vi "ConsolidatedLaunchingCode.vi"(8 "error in (no error)":errorcluster, 9 "Timeout (s)":i32, 11 "PullBack":bool) -> (0 "error out":errorcluster)   [LabVIEW 2013]
uses:
  <vilib>/Rock Robotics/WPI/CAN/Jaguar/SubVIs/WPI_CANJaguar_StatusSelect.ctl
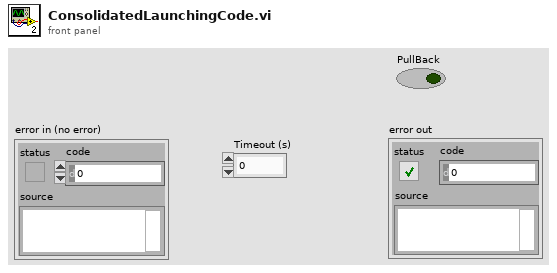
[diagram p1: front panel]
types:
  T1 = typedef "WPI_CANJaguar_StatusSelect.ctl" = enum16{"Output Percent VBus", "Output Voltage", "Bus Voltage", "Current", "Temperature", "Position", "Speed", "Limit Switches", "Faults", "Fault Counters", "Power Cycle"}
  T2 = typedef "WPI_MotorControlDeviceRef.ctl" = cluster{"DeviceStatus":errorcluster, "Type":enum16{"PWM", "CAN"}, "PWM":cluster{"Digital Module":T3, "PWM Channel":T4, "DeadBand":T5}, "CAN":cluster{"Device Number":u8, "Control Mode":T6, "Semaphore":T7, "Max Vout":dbl}, "Invert":bool, "TransformRef":T8, "InvTransformRef":T8}
  T3 = typedef "FPGA_TypedefDigitalModule.ctl" = enum16{"Digital Module 1", "Digital Module 2"}
  T4 = typedef "FPGA_DIOPWMChannel.ctl" = enum8{"PWM 1", "PWM 2", "PWM 3", "PWM 4", "PWM 5", "PWM 6", "PWM 7", "PWM 8", "PWM 9", "PWM 10", "Invalid"}
  T5 = typedef "WPI_PWMDeadband.ctl" = cluster{"Name":string, "maxPositivePwm":i32, "minPositivePwm":i32, "centerPwm":i32, "maxNegativePwm":i32, "minNegativePwm":i32, "angularRange":u16}
  T6 = typedef "WPI_CANJaguar_ControlMode.ctl" = enum8{"Percent VBus", "Current", "Speed", "Position", "Voltage"}
  T7 = typedef "Semaphore RefNum" = refnum<k1>
  T8 = typedef "WPI_PWMTransform_ConPane.ctl" = refnum<vi>
  T9 = typedef "WPI_CANJaguar_Status.ctl" = cluster{"Output Percent VBus":dbl, "Output Voltage":dbl, "Bus Voltage":dbl, "Current":dbl, "Temperature":dbl, "Position":dbl, "Speed":dbl, "Limits":cluster{"Forward Limit":bool, "Reverse Limit":bool, "Forward Soft Limit":bool, "Reverse Soft Limit":bool, "Sticky Forward Limit":bool, "Sticky Reverse Limit":bool, "Sticky Forward Soft Limit":bool, "Sticky Reverse Soft Limit":bool}, "Faults":cluster{"Current Fault":bool, "Temperature Fault":bool, "Bus Voltage Fault":bool, "Gate Driver Fault":bool, "Comm Fault":bool}, "Fault Counters":cluster{"Current Faults":u8, "Temperature Faults":u8, "Bus Voltage Faults":u8, "Gate Driver Faults":u8, "Comm Faults":u8, "CAN Status":u8, "CAN RX Errors":u8, "CAN TX Errors":u8}, "Power Cycle":bool}
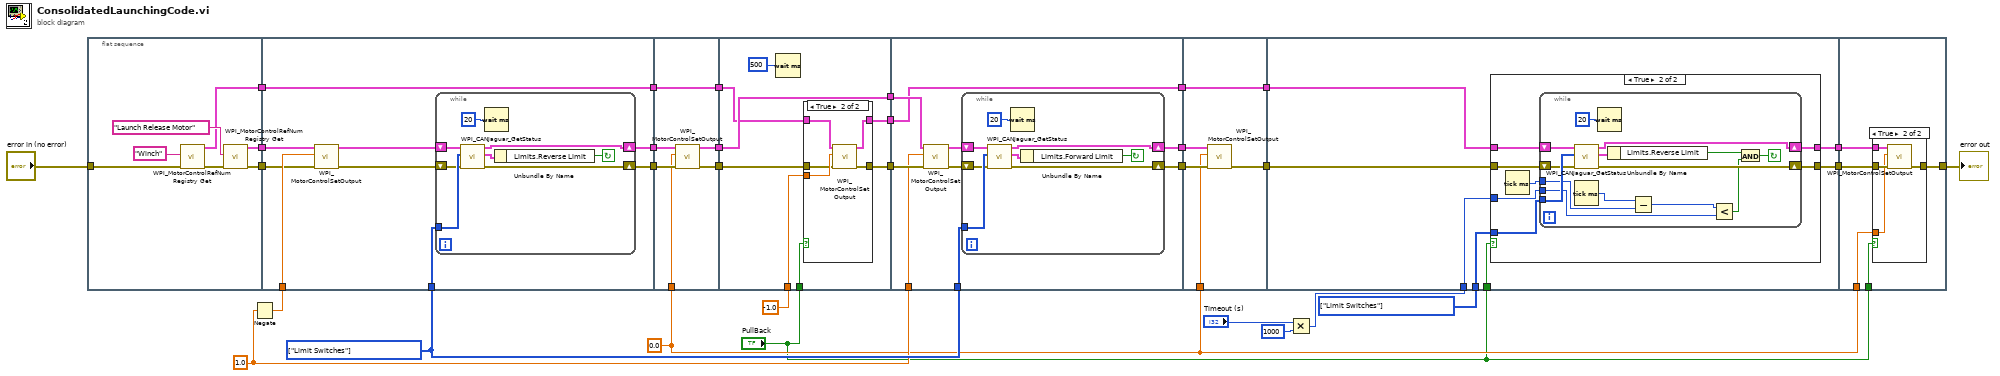
[diagram p0: block diagram]
diagram:
  w12 = T1[] [enum."Limit Switches"] items=["Output Percent VBus", "Output Voltage", "Bus Voltage", "Current", "Temperature", "Position", "Speed", "Limit Switches", "Faults", "Fault Counters", "Power Cycle"] ("Status Select")
  w5 = 0.0 ("Output")
  w17 = 1.0 ("Output")
  w19 = T1[] [enum."Limit Switches"] items=["Output Percent VBus", "Output Voltage", "Bus Voltage", "Current", "Temperature", "Position", "Speed", "Limit Switches", "Faults", "Fault Counters", "Power Cycle"] ("Status Select")
  n1 = flat-sequence {
    tunnel: "error in (no error)" -> [w35]
    tunnel: [w37] -> w31
    tunnel: [w36] -> w30
    tunnel: [w32] -> w2
    tunnel: w31 -> [w43]
    tunnel: w30 -> [w42]
    tunnel: [w46] -> w28
    tunnel: [w47] -> w29
    tunnel: w19 -> [w45]
    tunnel: w18 -> [w44]
    tunnel: [w39] -> w3
    tunnel: w2 -> [w39]
    tunnel: [w61] -> w27
    tunnel: [w60] -> w26
    tunnel: w29 -> [w58]
    tunnel: w28 -> [w59]
    tunnel: w5 -> [w57]
    tunnel: [w56] -> w4
    tunnel: w3 -> [w56]
    tunnel: w27 -> [w69]
    tunnel: [w69] -> w25
    tunnel: w26 -> [w63]
    tunnel: [w67] -> w24
    tunnel: -1.0 ("Output") -> [w66]
    tunnel: [w65] -> w9
    tunnel: w4 -> [w64]
    tunnel: "PullBack" -> [w62]
    tunnel: w25 -> [w85]
    tunnel: w24 -> [w84]
    tunnel: w19 -> [w80]
    tunnel: w17 -> [w83]
    tunnel: [w78] -> w23
    tunnel: [w79] -> w22
    tunnel: w9 -> [w77]
    tunnel: [w77] -> w8
    tunnel: w5 -> [w95]
    tunnel: w23 -> [w97]
    tunnel: w22 -> [w98]
    tunnel: [w96] -> w14
    tunnel: w8 -> [w94]
    tunnel: [w94] -> w7
    tunnel: w14 -> [w105]
    tunnel: w12 -> [w104]
    tunnel: w11 -> [w103]
    tunnel: [w102] -> w10
    tunnel: w7 -> [w101]
    tunnel: [w100] -> w6
    tunnel: "PullBack" -> [w99]
    tunnel: [w132] -> w21
    tunnel: w10 -> [w133]
    tunnel: w6 -> [w131]
    tunnel: w5 -> [w130]
    tunnel: "PullBack" -> [w129]
    frame #0 {
      n2 = call <vilib>:"WPI_MotorControlRefNum Registry Get.vi"("error in (no error)"=w35, "refnum name"="Winch") -> ("error out"=w34:errorcluster, "MotorControlDevRef"=w32:T2)  [unwired: 8 in]
      n3 = call <vilib>:"WPI_MotorControlRefNum Registry Get.vi"("error in (no error)"=w34, "refnum name"="Launch Release Motor") -> ("error out"=w36:errorcluster, "MotorControlDevRef"=w37:T2)  [unwired: 8 in]
    }
    frame #1 {
      n4 = call <vilib>:"WPI_MotorControlSetOutput.vi"("error in (no error)"=w42, "Output"=w44, "MotorControlDevRef"=w43) -> ("error out"=w40:errorcluster, "MotorControlDevRef"=w41:T2)  [unwired: 6 in, 1 out]
      n5 = while {
        shift-right: [w53] -> w47
        shift-left: w40 -> [w49]
        shift-right: [w52] -> w46
        shift-left: w41 -> [w50]
        tunnel: w45 -> [w51]
        stop <- w48 continue-if-true
        n6 = call <vilib>:"WPI_CANJaguar_GetStatus.vi"("error in (no error)"=w49, "Status Select"=w51, "CAN Jaguar Ref"=w50) -> ("error out"=w53:errorcluster, "Status"=w55:T9, "CAN Jaguar Ref Out"=w52:T2)  [unwired: 6 in]
        n7 = Wait (ms)(milliseconds to wait=u32 20) -> ()  [unwired: 1 out]
        n8 = Unbundle By Name(w55) -> ("Limits.Reverse Limit"=w48:bool)
      }
    }
    frame #2 {
      n9 = call <vilib>:"WPI_MotorControlSetOutput.vi"("error in (no error)"=w58, "Output"=w57, "MotorControlDevRef"=w59) -> ("error out"=w60:errorcluster, "MotorControlDevRef"=w61:T2)  [unwired: 6 in, 1 out]
    }
    frame #3 {
      n10 = Wait (ms)(milliseconds to wait=u32 500) -> ()  [unwired: 1 out]
      n11 = case shown="True" w62 {
        tunnel: [w70 w76] -> w67
        tunnel: w66 -> [_ w75]
        tunnel: [w71 w74] -> w65
        tunnel: w64 -> [w71 w73]
        tunnel: w63 -> [w70 w72]
        frame False {
        }
        frame True {
          n12 = call <vilib>:"WPI_MotorControlSetOutput.vi"("error in (no error)"=w72, "Output"=w75, "MotorControlDevRef"=w73) -> ("error out"=w76:errorcluster, "MotorControlDevRef"=w74:T2)  [unwired: 6 in, 1 out]
        }
      }
    }
    frame #4 {
      n13 = call <vilib>:"WPI_MotorControlSetOutput.vi"("error in (no error)"=w84, "Output"=w83, "MotorControlDevRef"=w85) -> ("error out"=w82:errorcluster, "MotorControlDevRef"=w81:T2)  [unwired: 6 in, 1 out]
      n14 = while {
        shift-right: [w91] -> w79
        shift-left: w82 -> [w87]
        shift-right: [w90] -> w78
        shift-left: w81 -> [w88]
        tunnel: w80 -> [w89]
        stop <- w86 continue-if-true
        n15 = call <vilib>:"WPI_CANJaguar_GetStatus.vi"("error in (no error)"=w87, "Status Select"=w89, "CAN Jaguar Ref"=w88) -> ("error out"=w91:errorcluster, "Status"=w93:T9, "CAN Jaguar Ref Out"=w90:T2)  [unwired: 6 in]
        n16 = Wait (ms)(milliseconds to wait=u32 20) -> ()  [unwired: 1 out]
        n17 = Unbundle By Name(w93) -> ("Limits.Forward Limit"=w86:bool)
      }
    }
    frame #5 {
      n18 = call <vilib>:"WPI_MotorControlSetOutput.vi"("error in (no error)"=w98, "Output"=w95, "MotorControlDevRef"=w97) -> ("error out"=w96:errorcluster)  [unwired: 6 in, 2 out]
    }
    frame #6 {
      n19 = case shown="True" w99 {
        tunnel: w105 -> [w106 w113]
        tunnel: w104 -> [_ w112]
        tunnel: w103 -> [_ w111]
        tunnel: [w106 w110] -> w102
        tunnel: w101 -> [w107 w109]
        tunnel: [w107 w108] -> w100
        frame False {
        }
        frame True {
          n20 = Tick Count (ms)() -> (millisecond timer value=w114:u32)
          n21 = while {
            shift-right: [w126] -> w110
            shift-left: w113 -> [w122]
            shift-right: [w125] -> w108
            shift-left: w109 -> [w123]
            tunnel: w112 -> [w124]
            tunnel: w114 -> [w117]
            tunnel: w111 -> [w115]
            stop <- w121 continue-if-true
            n22 = call <vilib>:"WPI_CANJaguar_GetStatus.vi"("error in (no error)"=w122, "Status Select"=w124, "CAN Jaguar Ref"=w123) -> ("error out"=w126:errorcluster, "Status"=w128:T9, "CAN Jaguar Ref Out"=w125:T2)  [unwired: 6 in]
            n23 = Tick Count (ms)() -> (millisecond timer value=w118:u32)
            n24 = Wait (ms)(milliseconds to wait=u32 20) -> ()  [unwired: 1 out]
            n25 = Unbundle By Name(w128) -> ("Limits.Reverse Limit"=w120:bool)
            n26 = Subtract(x=w118, y=w117) -> (x-y=w116:u32)
            n27 = Less?(x=w116, y=w115) -> (x < y?=w119:bool)
            n28 = And(x=w120, y=w119) -> (x .and. y?=w121:bool)
          }
        }
      }
    }
    frame #7 {
      n29 = case shown="True" w129 {
        tunnel: w133 -> [w134 w138]
        tunnel: [w134 w137] -> w132
        tunnel: w131 -> [_ w136]
        tunnel: w130 -> [_ w135]
        frame False {
        }
        frame True {
          n30 = call <vilib>:"WPI_MotorControlSetOutput.vi"("error in (no error)"=w138, "Output"=w135, "MotorControlDevRef"=w136) -> ("error out"=w137:errorcluster)  [unwired: 6 in, 2 out]
        }
      }
    }
  }
  n31 = Negate(x=w17) -> (-x=w18:dbl)
  n32 = Multiply(x="Timeout (s)", y=1000) -> (x*y=w11:i32)
  "error out" <- w21
